vi "TestHelper_CheckMessageHeaders.vi"(9 "Received Message":T1, 10 "Published Message":T1) -> (1 "Received Message Out":T1, 2 "Published Message Out":T1, 3 "Equal?":bool)   [LabVIEW 2017]
uses:
  <vilib>/addons/InsightCM/MessageBus/Base/controls/Message.ctl
  <vilib>/addons/InsightCM/MessageBus/Base/controls/MessageHeader.ctl
  <vilib>/addons/InsightCM/MessageBus/Base/controls/KeyValuePair.ctl
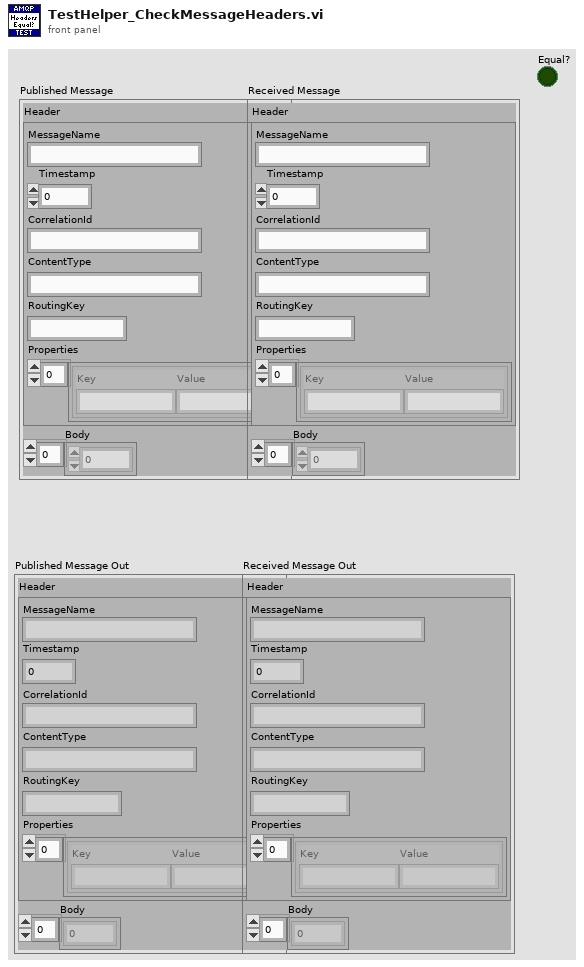
[diagram p1: front panel]
types:
  T1 = typedef "Message.ctl" = cluster{"Header":T2, "Body":u8[]}
  T2 = typedef "MessageHeader.ctl" = cluster{"MessageName":string, "Timestamp":i64, "CorrelationId":string, "ContentType":string, "RoutingKey":string, "Properties":T3[]}
  T3 = typedef "KeyValuePair.ctl" = cluster{"Key":string, "Value":string}
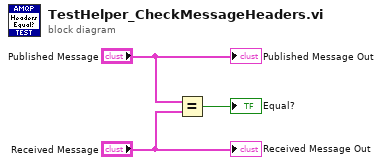
[diagram p0: block diagram]
diagram:
  n1 = Equal?(x="Published Message", y="Received Message") -> (x = y?=→"Equal?":bool)
  "Published Message Out" <- "Published Message"
  "Received Message Out" <- "Received Message"
